vi "ExpandDataPaths2.vi"(11 "Data File":path[](array[path])) -> (3 "Array":path[](array[path]))   [LabVIEW 2014]
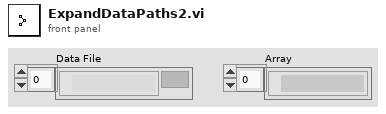
[diagram p1: front panel]
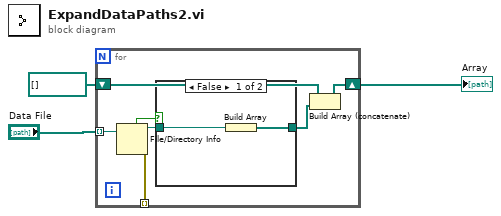
[diagram p0: block diagram]
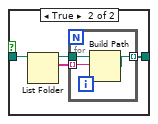
[diagram p2: hidden frame]
diagram:
  n1 = for {
    tunnel: "Data File" -> [w10] mode=indexing
    shift-right: [w5] -> w3
    shift-left: path[] [] -> [w7]
    tunnel: [w4] -> _ mode=indexing
    n2 = File/Directory Info(path=w10) -> (path out=w8:path, directory=w9:bool, error out=w4:errorcluster)  [unwired: 1 in, 4 out]
    n3 = case shown="False" w9 {
      tunnel: w8 -> [w12 w16]
      tunnel: [w11 w13] -> w6
      frame False {
        n4 = Build Array(w12) -> (w11:path[])
      }
      frame True {
        n5 = List Folder(path=w16) -> (path out=w15:path, filenames=w14:string[])  [unwired: 3 in, 2 out]
        n6 = for {
          tunnel: w15 -> [w19]
          tunnel: w14 -> [w18] mode=indexing
          tunnel: [w17] -> w13 mode=indexing
          n7 = Build Path(base path=w19, name or relative path=w18) -> (appended path=w17:path)
        }
      }
    }
    n8 = Build Array (concatenate)(w7, w6) -> (w5:path[])
  }
  "Array" <- w3
